vi "Is LV Object Default.vi"(1 "LabVIEW Object":refnum<class>) -> (0 "Is Default?":bool)   [LabVIEW 2020]
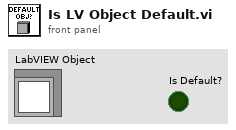
[diagram p1: front panel]
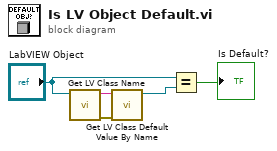
[diagram p0: block diagram]
diagram:
  n1 = call <vilib>:"Get LV Class Name.vi"("object"="LabVIEW Object") -> ("error out"=w5:errorcluster, "class name"=w4:string)  [unwired: 9 in]
  n2 = call <vilib>:"Get LV Class Default Value By Name.vi"("error in (no error)"=w5, "class name"=w4) -> ("object"=w1:refnum<class>)  [unwired: 8 in, 1 out]
  n3 = Equal?(x="LabVIEW Object", y=w1) -> (x = y?=→"Is Default?":bool)
